vi "状态机的使用(下).vi"() -> ()   [LabVIEW 2018]
panel:
  out "黄灯":bool
  out "绿灯":bool
  in  "枚举":enum16{"退出", "绿灯慢闪", "黄灯快闪", "灯全灭", "灯全亮", "等待"}(ring)
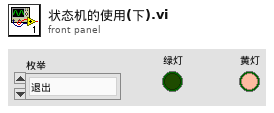
[diagram p1: front panel]
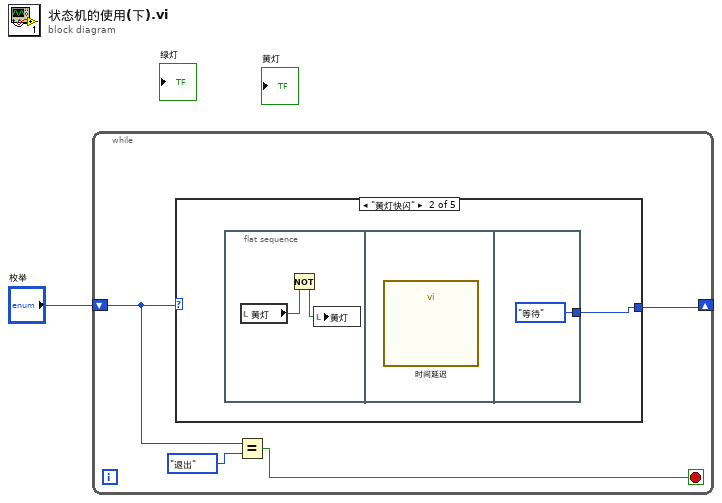
[diagram p0: block diagram]
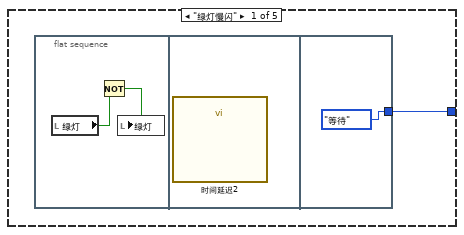
[diagram p2: hidden frame]
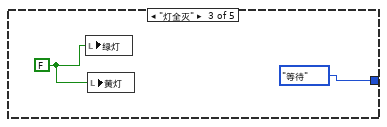
[diagram p3: hidden frame]
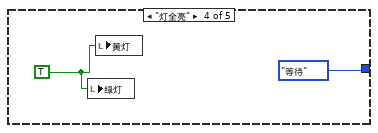
[diagram p4: hidden frame]
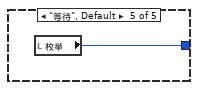
[diagram p5: hidden frame]
diagram:
  n1 = while {
    shift-right: [w5] -> _
    shift-left: "枚举" -> [w3]
    stop <- w2 stop-if-true
    n2 = case shown="\"黄灯快闪\"" w3 {
      tunnel: [w6 w10 enum16{"退出", "绿灯慢闪", "黄灯快闪", "灯全灭", "灯全亮", "等待"}."等待" ("枚举") enum16{"退出", "绿灯慢闪", "黄灯快闪", "灯全灭", "灯全亮", "等待"}."等待" ("枚举") w18] -> w5
      frame "绿灯慢闪" {
        n3 = flat-sequence {
          tunnel: [enum16{"退出", "绿灯慢闪", "黄灯快闪", "灯全灭", "灯全亮", "等待"}."等待" ("枚举")] -> w6
          frame #0 {
            n4 = local read "绿灯"() -> (w8:bool)
            n5 = Not(x=w8) -> (.not. x?=w7:bool)
            n6 = local write "绿灯"(w7) -> ()
          }
          frame #1 {
            n7 = call "时间延迟2"() -> ()  [unwired: 11 in, 1 out]
          }
          frame #2 {
          }
        }
      }
      frame "黄灯快闪" {
        n8 = flat-sequence {
          tunnel: [enum16{"退出", "绿灯慢闪", "黄灯快闪", "灯全灭", "灯全亮", "等待"}."等待" ("枚举")] -> w10
          frame #0 {
            n9 = local read "黄灯"() -> (w12:bool)
            n10 = Not(x=w12) -> (.not. x?=w11:bool)
            n11 = local write "黄灯"(w11) -> ()
          }
          frame #1 {
            n12 = call "时间延迟"() -> ()  [unwired: 11 in, 1 out]
          }
          frame #2 {
          }
        }
      }
      frame "灯全灭" {
        w15 = FALSE
        n13 = local write "绿灯"(w15) -> ()
        n14 = local write "黄灯"(w15) -> ()
      }
      frame "灯全亮" {
        w17 = TRUE
        n15 = local write "绿灯"(w17) -> ()
        n16 = local write "黄灯"(w17) -> ()
      }
      frame "等待", Default {
        n17 = local read "枚举"() -> (w18:enum16{"退出", "绿灯慢闪", "黄灯快闪", "灯全灭", "灯全亮", "等待"})
      }
    }
    n18 = Equal?(x=w3, y=enum16{"退出", "绿灯慢闪", "黄灯快闪", "灯全灭", "灯全亮", "等待"}."退出" ("枚举")) -> (x = y?=w2:bool)
  }
